vi "WebClient.vi"() -> (0 "error out":errorcluster, 3 "headers":string)   [LabVIEW 2021]
uses:
  <vilib>/httpClient/MultipartData.ctl
  <vilib>/httpClient/LabVIEWHTTPClient.lvlib
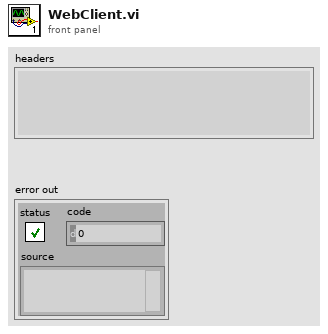
[diagram p1: front panel]
types:
  T1 = typedef "LabVIEWHTTPClient.lvlib/ClientHandle.ctl" = refnum<k1>
  T2 = typedef "LabVIEWHTTPClient.lvlib/MultipartData.ctl" = cluster{"Name":string, "Value":string, "File":path, "Filename":string, "MIME type":string}
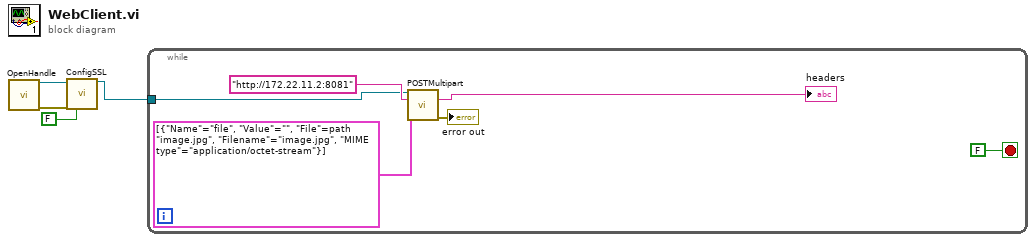
[diagram p0: block diagram]
diagram:
  n1 = call <vilib>:"OpenHandle.vi"() -> ("client handle out"=w1:T1, "error out"=w2:errorcluster)  [unwired: 14 in]
  n2 = call <vilib>:"ConfigSSL.vi"("client handle"=w1, "error in (no error)"=w2, "verify server (true)"=FALSE) -> ("client handle out"=w4:T1)  [unwired: 11 in, 1 out]
  n3 = while {
    tunnel: w4 -> [w5]
    stop <- FALSE stop-if-true
    n4 = call <vilib>:"POSTMultipart.vi"("client handle"=w5, "url"="http://172.22.11.2:8081", "data"=T2[] [{"Name"="file", "Value"="", "File"=path "/image.jpg", "Filename"="image.jpg", "MIME type"="application/octet-stream"}]) -> ("headers"=→"headers":string, "error out"=→"error out":errorcluster)  [unwired: 9 in, 2 out]
  }
